vi "Manual Test - Validate XML.vi"() -> ()   [LabVIEW 2020]
uses:
  <vilib>/Utility/xml.llb/Write to XML File(string).vi
  <vilib>/xml/Load XML File.vi
  <vilib>/xml/Close Reference(Node).vi
  <vilib>/xml/NI_XML.lvlib
  <resource>/objmgr/DOMUserDefRef.rc
panel:
  out "# Cluster Elements":i32
  out "Cluster Name":string
  out "Elements":string[](array[string])
  out "Element Name/Value":string[][](array[string])
  out "ClusterChildNodes":string[](array[string])
  out "XML":string
  in  "Process Data":T1={"VIPath"=path "C:/Data", "Menu Name"="Menu", "Selector Name"="Selector", "Time Stamp"=timestamp(3713362640.3208017 s since 1904-01-01)}
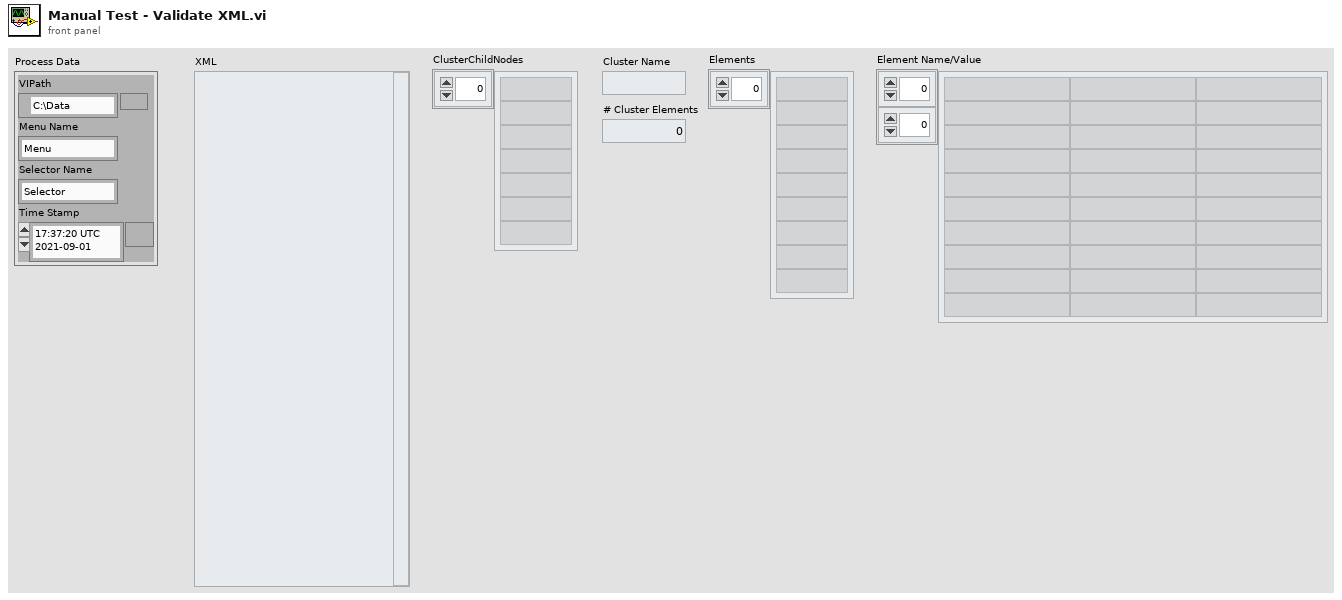
[diagram p1: front panel]
types:
  T1 = cluster{"VIPath":path, "Menu Name":string, "Selector Name":string, "Time Stamp":timestamp}
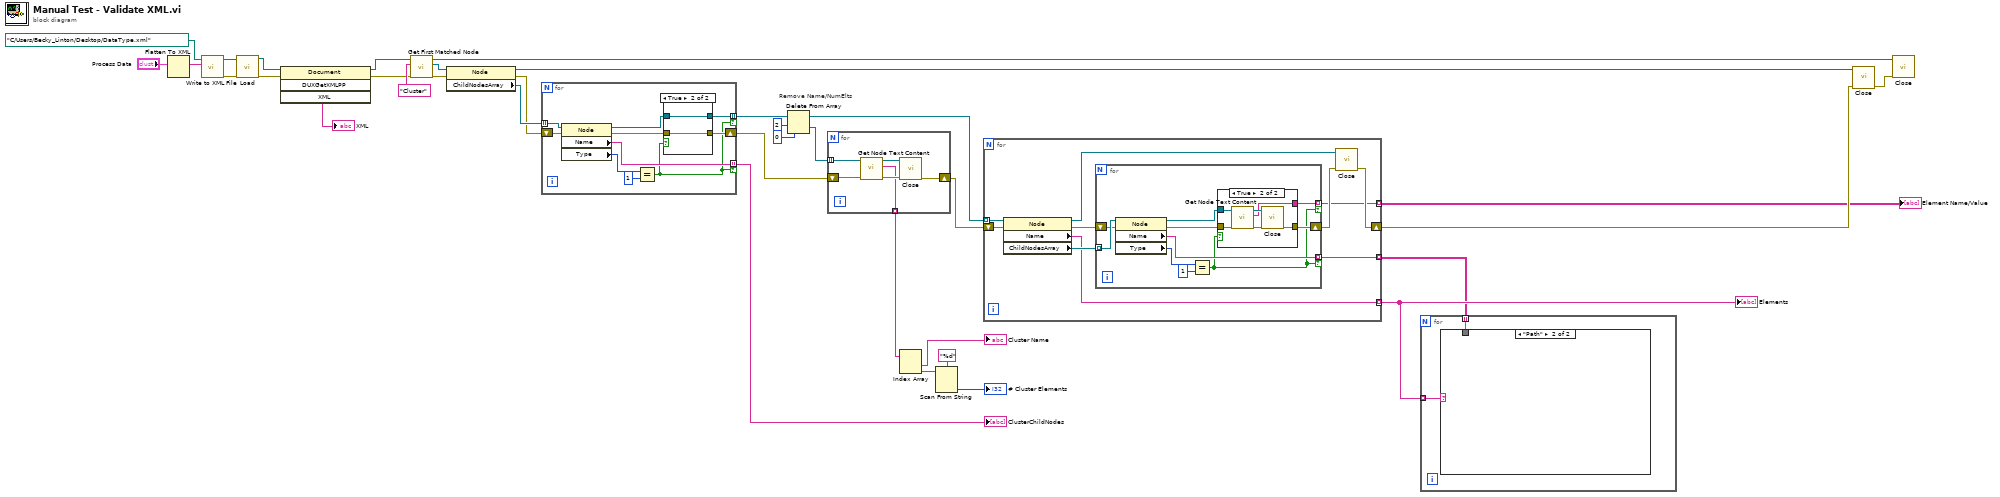
[diagram p0: block diagram]
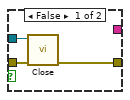
[diagram p3: hidden frame]
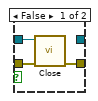
[diagram p4: hidden frame]
diagram:
  # "Remove Name/NumElts"
  n1 = Flatten To XML(6:"Process Data") -> (2:w30:string)
  n2 = call-poly <vilib>:"Write to XML File.vi"("XML Input"=w30, "XML File Path"=path "C:/Users/Becky_Linton/Desktop/DataType.xml") -> ("error out"=w32:errorcluster, "XML File Path(duplicate)"=w33:path)  [unwired: 7 in, 1 out]
  n3 = call-poly <vilib>:"Load.vi"("path to XML document"=w33, "error in (no error)"=w32) -> ("DOM document out"=w28:refnum<k20>, "error out"=w25:errorcluster)  [unwired: 11 in, 1 out]
  n4 = invoke class="Document" method="DUXGetXMLPP"(reference=w28, error in=w25) -> (reference out=w26:refnum<k20>, error out=w24:errorcluster, "XML"=→"XML":string)  [unwired: 2 in, 1 out]
  n5 = call <vilib>:"Get First Matched Node.vi"("error in (no error)"=w24, "XPath expression"="Cluster", "node in"=w26) -> ("error out"=w21:errorcluster, "node result"=w23:refnum<k20>, "node out"=w22:refnum<k20>)  [unwired: 6 in]
  n6 = property class="Node"(reference=w23, error in=w21) -> (reference out=w20:refnum<k20>, error out=w18:errorcluster, "ChildNodesArray"=w29:refnum<k20>[])
  n7 = for {
    tunnel: w29 -> [w45] mode=indexing
    tunnel: [w44] -> w17 mode=indexing if=w36
    shift-right: [w41] -> w10
    shift-left: w18 -> [w43]
    tunnel: [w37] -> w15 mode=indexing if=w36
    n8 = property class="Node"(reference=w45, error in=w43) -> (reference out=w40:refnum<k20>, error out=w42:errorcluster, "Name"=w44:string, "Type"=w39:i32)
    n9 = Equal?(x=w39, y=1) -> (x = y?=w36:bool)
    n10 = case shown="True" w36 {
      tunnel: w42 -> [w48 w49]
      tunnel: [w47 w49] -> w41
      tunnel: w40 -> [w46 w50]
      tunnel: [_ w50] -> w37
      frame False {
        n11 = call-poly <vilib>:"Close.vi"("error in (no error)"=w48, "node"=w46) -> ("error out"=w47:errorcluster)  [unwired: 7 in]
      }
      frame True {
      }
    }
  }
  "ClusterChildNodes" <- w17
  n12 = Delete From Array(array=w15, length=2, index=0) -> (deleted portion=w11:refnum<k20>[], array with subset deleted=w12:refnum<k20>[])
  n13 = for {
    tunnel: w11 -> [w55] mode=indexing
    shift-right: [w53] -> w9
    shift-left: w10 -> [w54]
    tunnel: [w51] -> w7 mode=indexing
    n14 = call <vilib>:"Get Node Text Content.vi"("error in (no error)"=w54, "node in"=w55) -> ("error out"=w52:errorcluster, "node text"=w51:string, "node out"=w56:refnum<k20>)  [unwired: 7 in]
    n15 = call-poly <vilib>:"Close.vi"("error in (no error)"=w52, "node"=w56) -> ("error out"=w53:errorcluster)  [unwired: 7 in]
  }
  n16 = Index Array(array=w7) -> (element #1=→"Cluster Name":string, element #2=w5:string)  [unwired: 2 in]
  n17 = Scan From String(format string="%d", input string=w5) -> (output 1=→"# Cluster Elements":i32)  [unwired: 3 in, 3 out]
  n18 = for {
    shift-right: [w60] -> w16
    shift-left: w9 -> [w66]
    tunnel: w12 -> [w63] mode=indexing
    tunnel: [w59] -> w1 mode=indexing
    tunnel: [w58] -> w8 mode=indexing
    tunnel: [w57] -> w2 mode=indexing
    n19 = property class="Node"(reference=w63, error in=w66) -> (reference out=w62:refnum<k20>, error out=w64:errorcluster, "Name"=w57:string, "ChildNodesArray"=w65:refnum<k20>[])
    n20 = for {
      tunnel: w65 -> [w76] mode=indexing
      tunnel: [w75] -> w59 mode=indexing if=w67
      shift-right: [w69] -> w61
      shift-left: w64 -> [w70]
      tunnel: [w68] -> w58 mode=indexing if=w67
      n21 = property class="Node"(reference=w76, error in=w70) -> (reference out=w72:refnum<k20>, error out=w71:errorcluster, "Name"=w75:string, "Type"=w74:i32)
      n22 = Equal?(x=w74, y=1) -> (x = y?=w67:bool)
      n23 = case shown="True" w67 {
        tunnel: w71 -> [w79 w84]
        tunnel: [w78 w82] -> w69
        tunnel: w72 -> [w77 w85]
        tunnel: [_ w80] -> w68
        frame False {
          n24 = call-poly <vilib>:"Close.vi"("error in (no error)"=w79, "node"=w77) -> ("error out"=w78:errorcluster)  [unwired: 7 in]
        }
        frame True {
          n25 = call <vilib>:"Get Node Text Content.vi"("error in (no error)"=w84, "node in"=w85) -> ("error out"=w83:errorcluster, "node text"=w80:string, "node out"=w81:refnum<k20>)  [unwired: 7 in]
          n26 = call-poly <vilib>:"Close.vi"("error in (no error)"=w83, "node"=w81) -> ("error out"=w82:errorcluster)  [unwired: 7 in]
        }
      }
    }
    n27 = call-poly <vilib>:"Close.vi"("error in (no error)"=w61, "node"=w62) -> ("error out"=w60:errorcluster)  [unwired: 7 in]
  }
  "Element Name/Value" <- w8
  "Elements" <- w2
  n28 = for {
    tunnel: w2 -> [w87] mode=indexing
    tunnel: w1 -> [w86] mode=indexing
    n29 = case shown="\"Path\"" w87 {
      tunnel: w86 -> [_ _]
      frame "False", Default {
      }
      frame "Path" {
      }
    }
  }
  n30 = call-poly <vilib>:"Close.vi"("error in (no error)"=w16, "node"=w20) -> ("error out"=w19:errorcluster)  [unwired: 7 in]
  n31 = call-poly <vilib>:"Close.vi"("error in (no error)"=w19, "node"=w22) -> ()  [unwired: 7 in, 1 out]
